vi "SMSD error handler.vi"(8 "error in (no error)":errorcluster, 9 "correct answer (OK)":T1, 10 "timed out?":bool, 11 "data":u8[](array[numeric])) -> (0 "error out":errorcluster)   [LabVIEW 2021, in "SMSD.lvclass"]
uses:
  SMSD.lvclass
  Data Unit/SMSD Data Unit/ERROR_OR_COMMANT_Type.ctl
  SMSD.lvclass/SMSD.ctl
  Data Unit/SMSD Data Unit/SMSD Data Unit.lvclass
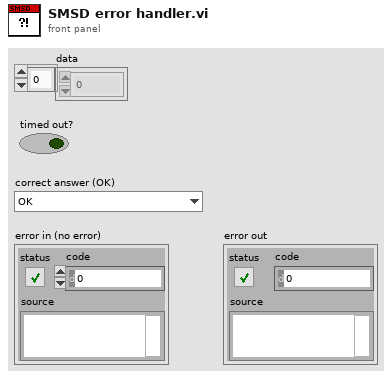
[diagram p1: front panel]
types:
  T1 = typedef "SMSD Data Unit.lvclass/ERROR_OR_COMMANT_Type.ctl" = enum8{"OK", "OK_ACCESS", "ERROR_ACCESS", "ERROR_ACCESS_TIMEOUT", "ERROR_XOR", "ERROR_NO_COMMAND", "ERROR_LEN", "ERROR_RANGE", "ERROR_WRITE", "ERROR_READ", "ERROR_PROGRAMS", "ERROR_WRITE_SETUP", "NO_NEXT", "END_PROGRAMS", "COMMAND_GET_STATUS_IN_EVENT", "COMMAND_GET_MODE", "COMMAND_GET_ABS_POS", "COMMAND_GET_EL_POS", "COMMAND_GET_SPEED", "COMMAND_GET_MIN_SPEED", "COMMAND_GET_MAX_SPEED", "COMMAND_GET_STACK", "STATUS_RELE_SET", "STATUS_RELE_CLR"}
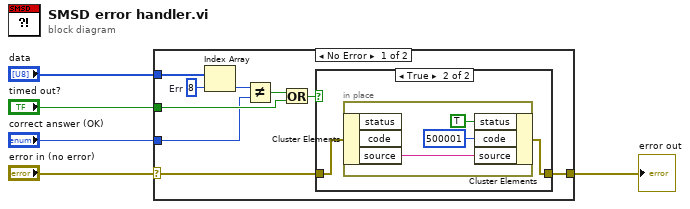
[diagram p0: block diagram]
diagram:
  n1 = case shown="No Error" "error in (no error)" {
    selector: "error in (no error)" -> [w7 w21]
    tunnel: "data" -> [w14 _]
    tunnel: "timed out?" -> [w10 _]
    tunnel: [w8 w21] -> w4
    tunnel: "correct answer (OK)" -> [w6 _]
    frame No Error {
      w13 = 8  # Err
      n2 = Index Array(array=w14, index=w13) -> (element=w12:u8)
      n3 = Not Equal?(x=w12, y=w6) -> (x != y?=w11:bool)
      n4 = Or(x=w11, y=w10) -> (x .or. y?=w9:bool)
      n5 = case shown="True" w9 {
        tunnel: [w15 w16] -> w8
        tunnel: w7 -> [w15 w17]
        frame False {
        }
        frame True {
          n6 = in-place {
            n7 = in-place-cluster #1(w17) -> ("source"=w18:string)  [unwired: 2 out]
            n8 = in-place-cluster #1("status"=TRUE, "code"=500001, "source"=w18) -> (w16:errorcluster)
          }
        }
      }
    }
    frame Error {
    }
  }
  "error out" <- w4
